vi "ProcessControl.vi"(11 "Row":i32) -> (3 "Process":T1)   [LabVIEW 2013]
uses:
  Control/SystemProcess.ctl
  Control/Buffer.vi
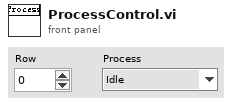
[diagram p1: front panel]
types:
  T1 = typedef "SystemProcess.ctl" = enum16{"Idle", "SystemInit", "SpecialEvent", "Barcode(SN)", "TestInitialize", "Test", "Stop", "SaveTestData", "Exit"}
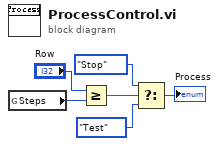
[diagram p0: block diagram]
diagram:
  n1 = global read "Buffer.vi" "Steps"() -> (w6:i32)
  n2 = Greater Or Equal?(x="Row", y=w6) -> (x >= y?=w2:bool)
  n3 = Select(t=SystemProcess."Stop" ("SystemProcess"), s=w2, f=SystemProcess."Test") -> (s? t:f=→"Process":T1)
